vi "System_ID.vi"(4 "Input Order":i32=1, 5 "Output Order":i32=2, 6 "error in (no error)":errorcluster, 8 "Input Array":dbl[](array[numeric]), 9 "Output Array":dbl[](array[numeric])) -> (0 "error out":errorcluster, 1 "Output vs Model":dbl[][](graph), 2 "Resultant Parameters":T1, 3 "RMSE":dbl format="%0.2f")   [LabVIEW 2020]
uses:
  <vilib>/Analysis/Matrix/Datatypes/RealMatrix.ctl
  <vilib>/Analysis/baseanly.llb/Real A x B.vi
  <vilib>/Analysis/_algsub.llb/Real PseudoInverse Matrix.vi
  <vilib>/Analysis/Matrix/Numeric/Conversions/Array To Matrix - RA.vi
  <vilib>/Analysis/Matrix/Numeric/Conversions/Matrix To Array - RM.vi
  <vilib>/Analysis/Matrix/Numeric/Conversions/Array To Matrix - RA2.vi
  <vilib>/Analysis/Matrix/NI_Matrix.lvlib
  <vilib>/Analysis/NI_AALPro.lvlib
  <vilib>/Analysis/NI_AALBase.lvlib
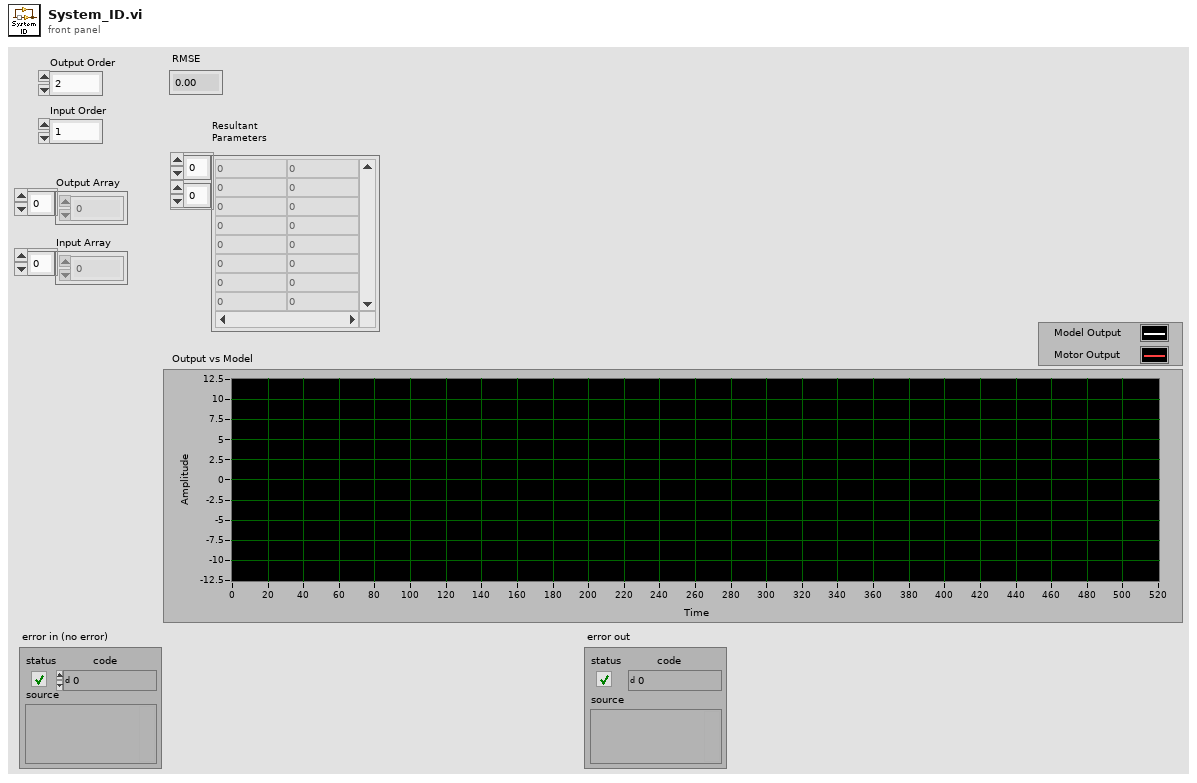
[diagram p1: front panel]
types:
  T1 = typedef "NI_Matrix.lvlib/RealMatrix.ctl" = dbl[][]
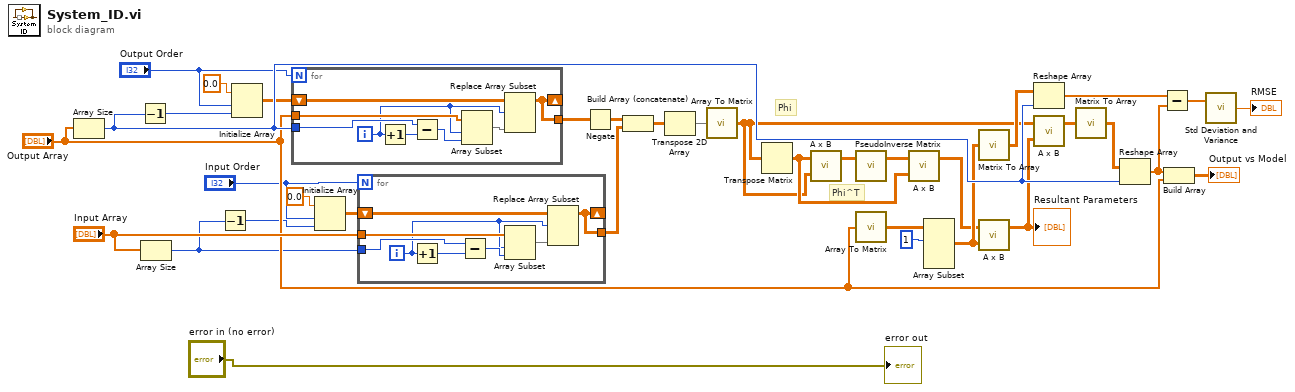
[diagram p0: block diagram]
diagram:
  # "Phi^T"
  # "Phi"
  n1 = Array Size(array="Output Array") -> (size(s)=w33:i32)
  n2 = Decrement(x=w33) -> (x-1=w7:i32)
  n3 = Array Size(array="Input Array") -> (size(s)=w10:i32)
  n4 = Decrement(x=w10) -> (x-1=w6:i32)
  n5 = Initialize Array(0.0 ("element"), "Output Order", w7) -> (w3:dbl[][])
  n6 = for {
    N: "Output Order" -> [_]
    tunnel: "Output Array" -> [w42]
    tunnel: w33 -> [w43]
    shift-right: [w36] -> _
    shift-left: w3 -> [w39]
    tunnel: [w36] -> w29
    i -> [w38]
    n7 = Increment(x=w38) -> (x+1=w37:i32)
    n8 = Subtract(x=w43, y=w37) -> (x-y=w41:i32)
    n9 = Array Subset(array=w42, index=w38, length=w41) -> (w40:dbl[])
    n10 = Replace Array Subset(array=w39, new element=w40, index (row)=w38) -> (w36:dbl[][])  [unwired: 1 in]
  }
  n11 = Initialize Array(0.0 ("element"), "Input Order", w6) -> (w5:dbl[][])
  n12 = for {
    N: "Input Order" -> [_]
    tunnel: "Input Array" -> [w50]
    tunnel: w10 -> [w51]
    shift-right: [w44] -> _
    shift-left: w5 -> [w47]
    tunnel: [w44] -> w11
    i -> [w46]
    n13 = Increment(x=w46) -> (x+1=w45:i32)
    n14 = Subtract(x=w51, y=w45) -> (x-y=w49:i32)
    n15 = Array Subset(array=w50, index=w46, length=w49) -> (w48:dbl[])
    n16 = Replace Array Subset(array=w47, new element=w48, index (row)=w46) -> (w44:dbl[][])  [unwired: 1 in]
  }
  n17 = Negate(x=w29) -> (-x=w30:dbl[][])
  n18 = Build Array (concatenate)(w30, w11) -> (w12:dbl[][])
  n19 = Transpose 2D Array(2D array=w12) -> (transposed array=w13:dbl[][])
  n20 = call-poly <vilib>:"Array To Matrix.vi"("Real 2D Array"=w13) -> ("Real Matrix"=w18:T1)
  n21 = Transpose Matrix(1:w18) -> (0:w19:T1)
  n22 = call-poly <vilib>:"A x B.vi"("B"=w18, "A"=w19) -> ("A x B"=w14:T1)  [unwired: 1 out]
  n23 = call-poly <vilib>:"PseudoInverse Matrix.vi"("Input Matrix"=w14) -> ("PseudoInverse Matrix"=w15:T1)  [unwired: 1 in, 1 out]
  n24 = call-poly <vilib>:"Array To Matrix.vi"("Real 1D Array"="Output Array") -> ("Real Matrix (Column Vector)"=w21:T1)
  n25 = call-poly <vilib>:"A x B.vi"("B"=w19, "A"=w15) -> ("A x B"=w16:T1)  [unwired: 1 out]
  n26 = Array Subset(array=w21, index (row)=1 ("row N")) -> (w31:T1)  [unwired: 3 in]
  n27 = call-poly <vilib>:"Matrix To Array.vi"("Real Matrix"=w31) -> ("Real 2D Array"=w32:dbl[][])
  n28 = call-poly <vilib>:"A x B.vi"("B"=w31, "A"=w16) -> ("A x B"=w17:T1)  [unwired: 1 out]
  "Resultant Parameters" <- w17
  n29 = Reshape Array(w32, w33) -> (w34:dbl[])
  n30 = call-poly <vilib>:"A x B.vi"("B"=w17, "A"=w18) -> ("A x B"=w22:T1)  [unwired: 1 out]
  n31 = call-poly <vilib>:"Matrix To Array.vi"("Real Matrix"=w22) -> ("Real 2D Array"=w23:dbl[][])
  n32 = Reshape Array(w23, w33) -> (w26:dbl[])
  n33 = Subtract(x=w34, y=w26) -> (x-y=w27:dbl[])
  n34 = Build Array(w26, "Output Array") -> (→"Output vs Model":dbl[][])
  n35 = call <vilib>:"Std Deviation and Variance.vi"("X"=w27) -> ("standard deviation"=→"RMSE":dbl)  [unwired: 1 in, 2 out]
  "error out" <- "error in (no error)"
